vi "mWmotor_set_motor_para.vi"(8 "error in (no error)":errorcluster, 10 "VISA resource name":refnum<visa-resource-name>, 11 "configuration file path":path=path "E:/E1039/Microwave/config.ini") -> (0 "error out":errorcluster, 1 "Intercept":dbl, 2 "Slope":dbl, 3 "VISA resource name out":refnum<visa-resource-name>)   [LabVIEW 2019]
uses:
  <vilib>/Utility/config.llb/Read Key (Double).vi
  <vilib>/Utility/config.llb/NI_LVConfig.lvlib
panel:
  in  "milliseconds to wait":u32=100
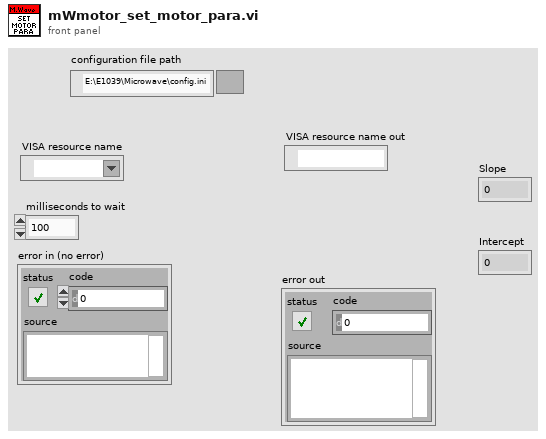
[diagram p1: front panel]
types:
  T1 = typedef "NI_LVConfig.lvlib/Config Data RefNum.ctl" = refnum<k1>
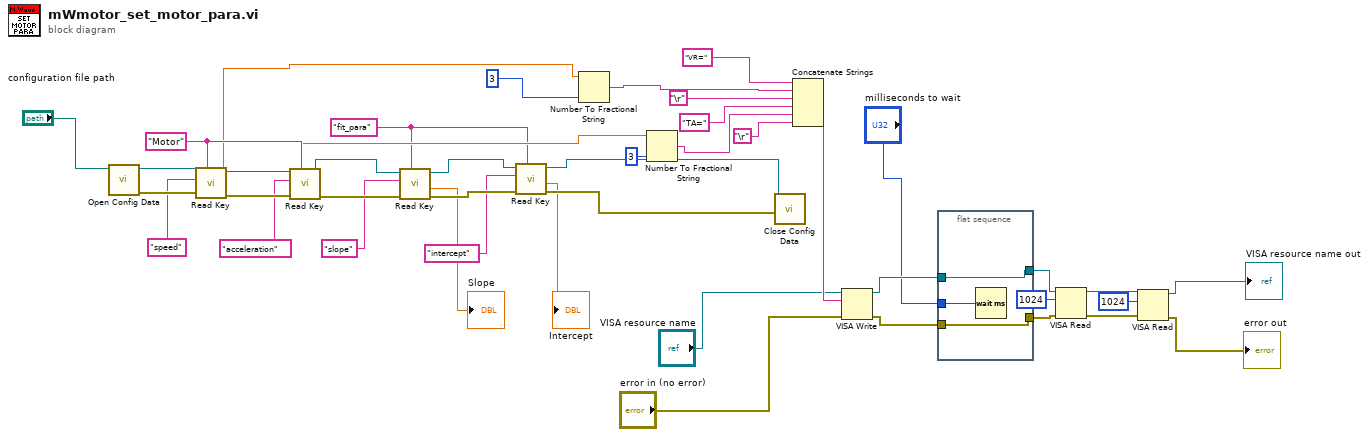
[diagram p0: block diagram]
diagram:
  w6 = "fit_para" ("section")
  w39 = "Motor" ("section")
  n1 = call <vilib>:"Open Config Data.vi"("configuration file path"="configuration file path") -> ("error out"=w40:errorcluster, "refnum"=w43:T1)  [unwired: 8 in, 1 out]
  n2 = call-poly <vilib>:"Read Key.vi"("section"=w39, "error in (no error)"=w40, "key"="speed", "refnum"=w43) -> ("error out"=w41:errorcluster, "value"=w1:dbl, "refnum out"=w42:T1)  [unwired: 4 in, 1 out]
  n3 = call-poly <vilib>:"Read Key.vi"("section"=w39, "error in (no error)"=w41, "key"="acceleration", "refnum"=w42) -> ("error out"=w12:errorcluster, "value"=w27:dbl, "refnum out"=w11:T1)  [unwired: 4 in, 1 out]
  n4 = call-poly <vilib>:"Read Key.vi"("section"=w6, "error in (no error)"=w12, "key"="slope", "refnum"=w11) -> ("error out"=w8:errorcluster, "value"=→"Slope":dbl, "refnum out"=w10:T1)  [unwired: 4 in, 1 out]
  n5 = call-poly <vilib>:"Read Key.vi"("section"=w6, "error in (no error)"=w8, "key"="intercept", "refnum"=w10) -> ("error out"=w7:errorcluster, "value"=→"Intercept":dbl, "refnum out"=w9:T1)  [unwired: 4 in, 1 out]
  n6 = Number To Fractional String(number=w1, precision (6)=i16 3) -> (F-format string=w14:string)  [unwired: 2 in]
  n7 = Number To Fractional String(number=w27, precision (6)=i16 3) -> (F-format string=w16:string)  [unwired: 2 in]
  n8 = call <vilib>:"Close Config Data.vi"("error in (no error)"=w7, "refnum"=w9) -> ()  [unwired: 8 in, 2 out]
  n9 = Concatenate Strings("VR=" ("string"), w14, "\r", "TA=" ("string"), w16, "\r") -> (w35:string)
  n10 = VISA Write(VISA resource name="VISA resource name", write buffer=w35, error in (no error)="error in (no error)") -> (VISA resource name out=w31:refnum<visa-resource-name>, error out=w32:errorcluster)  [unwired: 1 out]
  n11 = flat-sequence {
    tunnel: [w46] -> w24
    tunnel: w32 -> [w46]
    tunnel: [w45] -> w26
    tunnel: w31 -> [w45]
    tunnel: "milliseconds to wait" -> [w44]
    frame #0 {
      n12 = Wait (ms)(milliseconds to wait=w44) -> ()  [unwired: 1 out]
    }
  }
  n13 = VISA Read(VISA resource name=w26, byte count=u32 1024, error in (no error)=w24) -> (VISA resource name out=w23:refnum<visa-resource-name>, error out=w22:errorcluster)  [unwired: 2 out]
  n14 = VISA Read(VISA resource name=w23, byte count=u32 1024, error in (no error)=w22) -> (VISA resource name out=→"VISA resource name out":refnum<visa-resource-name>, error out=→"error out":errorcluster)  [unwired: 2 out]
